vi "ex_unMakeNamesGeneric.vi"(8 "error in (no error)":errorcluster, 9 "Renamed Controls":string[][](array[string]), 11 "VI refnum":refnum<vi>) -> (0 "error out":errorcluster)   [LabVIEW 2020]
doc: "Changes the names of the controls listed in the Renamed Controls array."
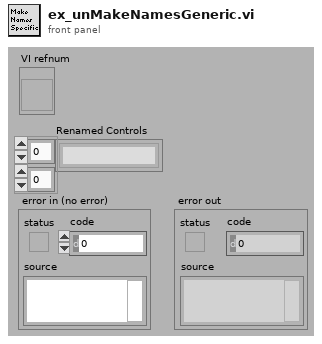
[diagram p1: front panel]
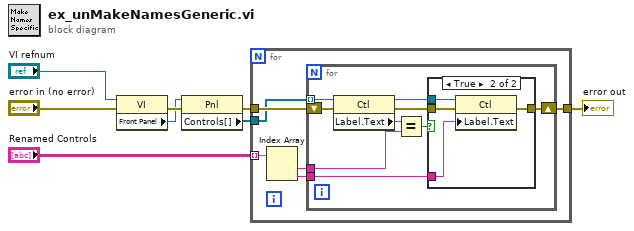
[diagram p0: block diagram]
diagram:
  n1 = property class="VI"(reference="VI refnum", error in="error in (no error)") -> (error out=w5:errorcluster, "Front Panel"=w3:refnum<vi>)  [unwired: 1 out]
  n2 = property class="Pnl"(reference=w3, error in=w5) -> (error out=w7:errorcluster, "Controls[]"=w4:refnum<vi>[])  [unwired: 1 out]
  n3 = for {
    tunnel: "Renamed Controls" -> [w13] mode=indexing
    tunnel: w4 -> [w10]
    tunnel: [w14] -> w6
    tunnel: w7 -> [w11]
    n4 = Index Array(array=w13) -> (element #1=w9:string, element #2=w12:string)  [unwired: 2 in]
    n5 = for {
      tunnel: w10 -> [w23] mode=indexing
      tunnel: w9 -> [w16]
      shift-right: [w18] -> w14
      shift-left: w11 -> [w17]
      tunnel: w12 -> [w15]
      n6 = property class="Ctl"(reference=w23, error in=w17) -> (reference out=w21:refnum<vi>, error out=w19:errorcluster, "Label.Text"=w22:string)
      n7 = Equal?(x=w22, y=w16) -> (x = y?=w20:bool)
      n8 = case shown="True" w20 {
        tunnel: w21 -> [_ w28]
        tunnel: w15 -> [_ w25]
        tunnel: w19 -> [w24 w27]
        tunnel: [w24 w26] -> w18
        frame False {
        }
        frame True {
          n9 = property class="Ctl"(reference=w28, error in=w27, "Label.Text"=w25) -> (error out=w26:errorcluster)  [unwired: 1 out]
        }
      }
    }
  }
  "error out" <- w6
